vi "Write Num.vi"(8 "error in (no error)":errorcluster, 10 "Ctl Refnum":refnum<vi>, 11 "Worksheet Reference":refnum<k7>) -> (0 "error out":errorcluster)   [LabVIEW 2015]
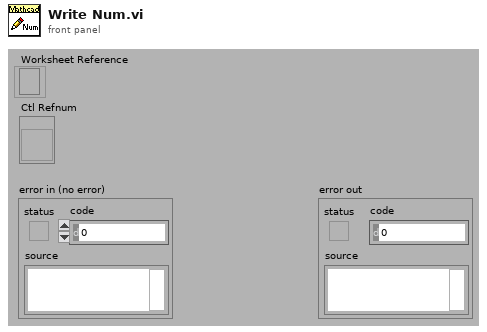
[diagram p1: front panel]
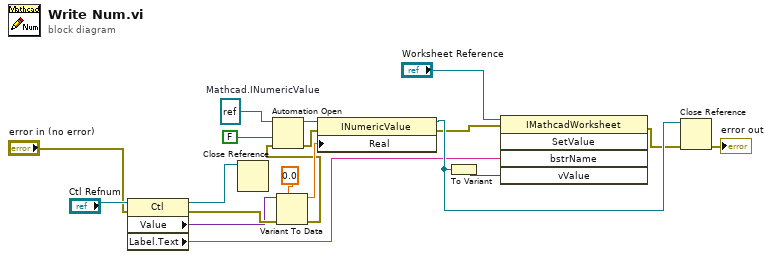
[diagram p0: block diagram]
diagram:
  w10 = refnum<k7> refnum  # Mathcad.INumericValue
  n1 = property class="Ctl"(reference="Ctl Refnum", error in="error in (no error)") -> (reference out=w5:refnum<vi>, error out=w13:errorcluster, "Value"=w12:variant, "Label.Text"=w1:string)
  n2 = Close Reference(reference=w5) -> ()  [unwired: 1 in, 1 out]
  n3 = Variant To Data(error in=w13, type=0.0, Variant=w12) -> (data=w11:dbl, error out=w2:errorcluster)
  n4 = Automation Open(error in (no error)=w2, Automation Refnum=w10, 9:FALSE ("open new instance")) -> (Automation Refnum=w18:refnum<k7>, error out=w17:errorcluster)  [unwired: 1 in]
  n5 = property class="INumericValue"(reference=w18, error in=w17, "Real"=w11) -> (reference out=w15:refnum<k7>, error out=w4:errorcluster)
  n6 = To Variant(anything=w15) -> (Variant=w16:variant)
  n7 = invoke class="IMathcadWorksheet" method="SetValue"(reference="Worksheet Reference", error in=w4, "bstrName"=w1, "vValue"=w16) -> (error out=w14:errorcluster)  [unwired: 1 in, 4 out]
  n8 = Close Reference(reference=w15, error in (no error)=w14) -> (error out=→"error out":errorcluster)
